vi "Read.vi"(0 "reference in":refnum<class "ConfigJSON.lvclass">, 5 "Type and Defaults":variant, 7 "Name":string, 11 "error in (no error)":errorcluster) -> (4 "reference out":refnum<class "ConfigJSON.lvclass">, 6 "Data":variant, 8 "Name dub":string, 15 "error out":errorcluster)   [LabVIEW 2019, in "ConfigJSON.lvclass"]
uses:
  ConfigJSON.lvclass
  ConfigJSON.lvclass/ConfigJSON.ctl
  <vilib>/addons/_JKI.lib/Serialization/JSON/JKI JSON Serialization.lvlib
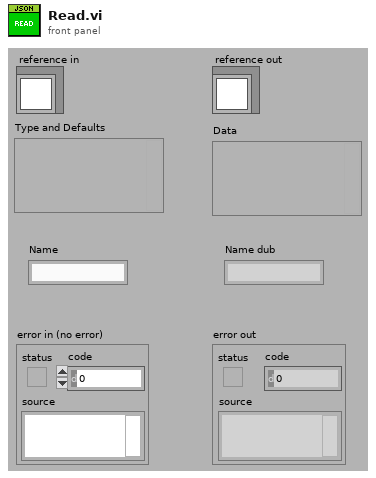
[diagram p1: front panel]
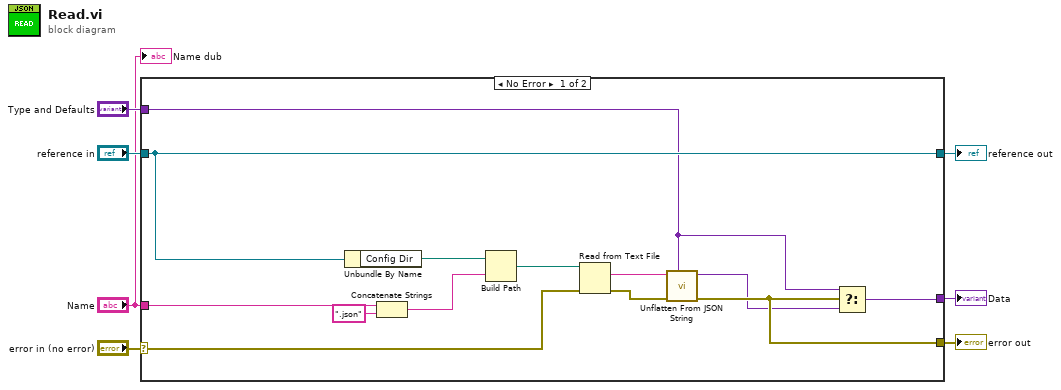
[diagram p0: block diagram]
diagram:
  n1 = case shown="No Error" "error in (no error)" {
    selector: "error in (no error)" -> [w19 w22]
    tunnel: [w9 w21] -> w7
    tunnel: "reference in" -> [w20 w23]
    tunnel: [w12 w22] -> w4
    tunnel: "Type and Defaults" -> [w11 w21]
    tunnel: [w20 w23] -> w2
    tunnel: "Name" -> [w17 _]
    frame No Error {
      n2 = Unbundle By Name(w20) -> ("Config Dir"=w18:path)
      n3 = Concatenate Strings(w17, ".json" ("string")) -> (w15:string)
      n4 = Build Path(base path=w18, name or relative path=w15) -> (appended path=w14:path)
      n5 = Read from Text File(file (use dialog)=w14, error in=w19) -> (text=w13:string, error out=w8:errorcluster)  [unwired: 2 in, 2 out]
      n6 = call <vilib>:"Unflatten From JSON String.vi"("Type and Defaults"=w11, "error in (no error)"=w8, "JSON String"=w13) -> ("error out"=w12:errorcluster, "Variant"=w10:variant)  [unwired: 7 in]
      n7 = Select(t=w11, s=w12, f=w10) -> (s? t:f=w9:variant)
    }
    frame Error {
    }
  }
  "error out" <- w4
  "reference out" <- w2
  "Data" <- w7
  "Name dub" <- "Name"
